vi "실습 2-8 문자열함수.vi"() -> ()   [LabVIEW 2014]
panel:
  out "숫자":dbl
  out "문자열 3":string="12.345"
  out "길이":i32
  out "문자열 2":string="12.345"
  in  "문자열":string="12.345"
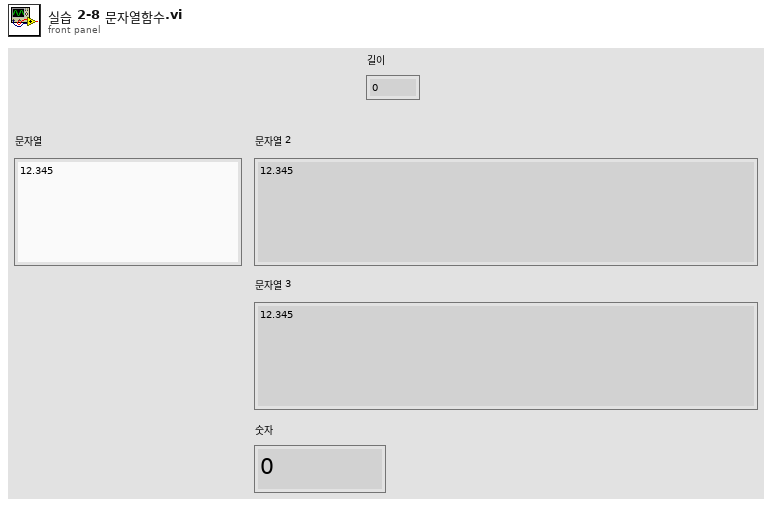
[diagram p1: front panel]
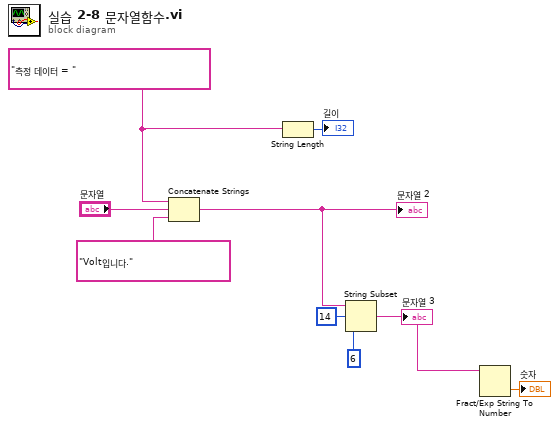
[diagram p0: block diagram]
diagram:
  w7 = "측정 데이터 = " ("문자열")
  n1 = Concatenate Strings(w7, "문자열", "Volt입니다." ("문자열")) -> (w5:string)
  "문자열 2" <- w5
  n2 = String Length(string=w7) -> (length=→"길이":i32)
  n3 = String Subset(string=w5, offset (0)=14 ("오프셋(0)"), length (rest)=6 ("길이(나머지)")) -> (substring=w2:string)
  "문자열 3" <- w2
  n4 = Fract/Exp String To Number(string=w2) -> (number=→"숫자":dbl)  [unwired: 3 in, 1 out]
